vi "rejestr z wpisem równoległym.vi"(8 "Wejście danych":bool[](array[boolean]), 11 "Switch":bool) -> (0 "Wyjście danych":bool[](array[boolean]), 4 "zliczenia wyjścia":u32, 5 "zalicenia wejścia":u32)   [LabVIEW 2020]
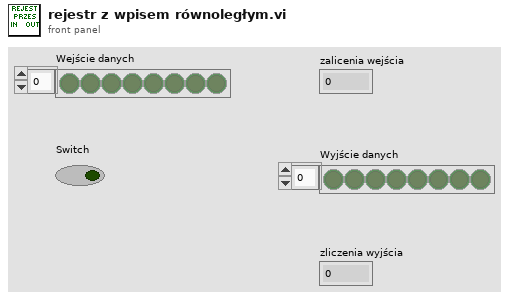
[diagram p1: front panel]
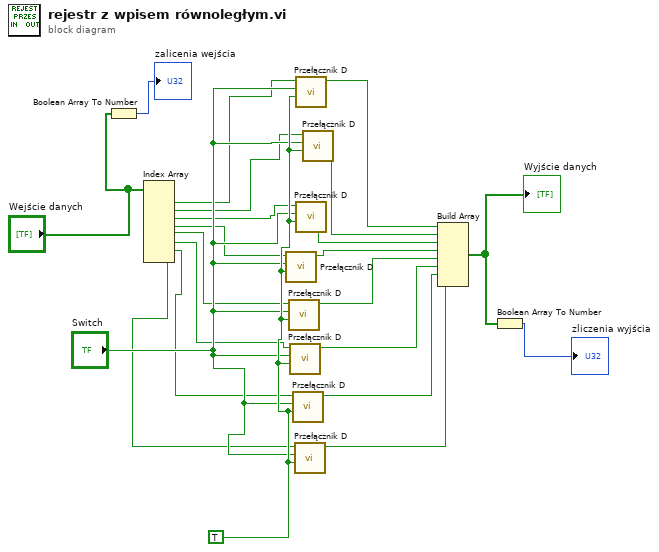
[diagram p0: block diagram]
diagram:
  w22 = TRUE
  n1 = Boolean Array To Number(Boolean array="Wejście danych") -> (number=→"zalicenia wejścia":u32)
  n2 = Index Array(array="Wejście danych") -> (element #1=w5:bool, element #2=w7:bool, element #3=w20:bool, element #4=w10:bool, element #5=w12:bool, element #6=w14:bool, element #7=w15:bool, element #8=w17:bool)  [unwired: 8 in]
  n3 = call "Przełącznik D.vi"("R"=w22, "C"="Switch", "D"=w10) -> ("Q"=w9:bool)  [unwired: 7 in, 1 out]
  n4 = call "Przełącznik D.vi"("R"=w22, "C"="Switch", "D"=w12) -> ("Q"=w11:bool)  [unwired: 7 in, 1 out]
  n5 = call "Przełącznik D.vi"("R"=w22, "C"="Switch", "D"=w14) -> ("Q"=w13:bool)  [unwired: 7 in, 1 out]
  n6 = call "Przełącznik D.vi"("R"=w22, "C"="Switch", "D"=w15) -> ("Q"=w16:bool)  [unwired: 7 in, 1 out]
  n7 = call "Przełącznik D.vi"("R"=w22, "C"="Switch", "D"=w17) -> ("Q"=w18:bool)  [unwired: 7 in, 1 out]
  n8 = call "Przełącznik D.vi"("R"=w22, "C"="Switch", "D"=w5) -> ("Q"=w6:bool)  [unwired: 7 in, 1 out]
  n9 = call "Przełącznik D.vi"("R"=w22, "C"="Switch", "D"=w20) -> ("Q"=w8:bool)  [unwired: 7 in, 1 out]
  n10 = call "Przełącznik D.vi"("R"=w22, "C"="Switch", "D"=w7) -> ("Q"=w19:bool)  [unwired: 7 in, 1 out]
  n11 = Build Array(w6, w19, w8, w9, w11, w13, w16, w18) -> (w2:bool[])
  "Wyjście danych" <- w2
  n12 = Boolean Array To Number(Boolean array=w2) -> (number=→"zliczenia wyjścia":u32)
